vi "Set Function None.vi"(0 "VISA resource name":refnum<visa-resource-name>, 5 "Channel":u16(ring) items=["A1"=0, "A2"=1, "A3"=2, "A4"=3, "A5"=4, "A6"=5, "A7"=6, "A8"=7, "A9"=8, "A10"=9, "K1"=200, "K2"=201, "K3"=202, "K4"=203, "FA1"=204, "FA2"=205, "FA3"=206, "FA4"=207], 11 "error in (no error)":errorcluster) -> (4 "VISA resource name out":refnum<visa-resource-name>, 15 "error out":errorcluster)   [LabVIEW 2017, in "Sefram DAS220.lvlib"]
doc: "No function"
uses:
  <instrlib>/Sefram DAS220/Sefram DAS220.lvlib
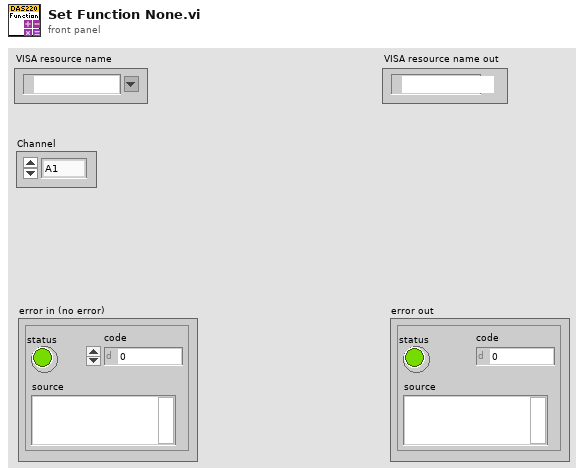
[diagram p1: front panel]
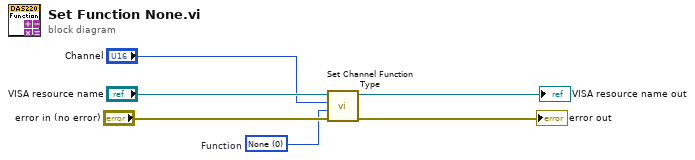
[diagram p0: block diagram]
diagram:
  w2 = u16 0 items=["None", "Change Unit", "aX+b", "a abs(X)+b", "aX2+bX+c", "a ln(X)+b", "a sqrt(dX+c)+b", "a exp(cX)+b", "a(1/X)+b"]  # Function
  n1 = call <instrlib>:"Set Channel Function Type.vi"("error in (no error)"="error in (no error)", "Function"=w2, "Channel"="Channel", "VISA resource name"="VISA resource name") -> ("error out"=→"error out":errorcluster, "VISA resource name out"=→"VISA resource name out":refnum<visa-resource-name>)  [unwired: 6 in]
